vi "Host - LED encode (SubVI).vi"(7 "Address":u8, 9 "Dim Ctrl":u8, 10 "led":bool) -> (2 "string":string, 3 "Command":string)   [LabVIEW 2021]
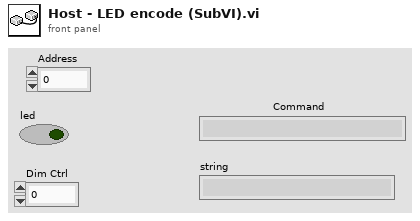
[diagram p1: front panel]
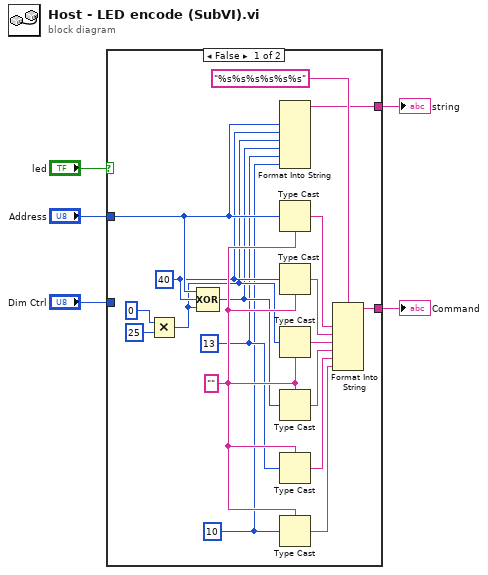
[diagram p0: block diagram]
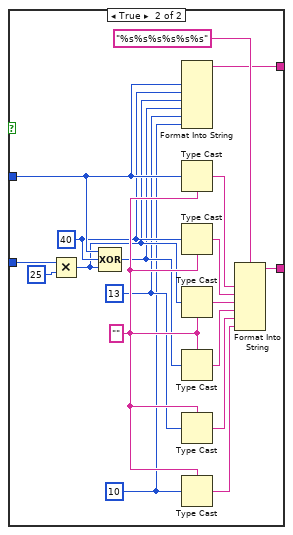
[diagram p2: hidden frame]
diagram:
  n1 = case shown="False" "led" {
    tunnel: "Dim Ctrl" -> [_ w41]
    tunnel: "Address" -> [w12 w30]
    tunnel: [w14 w31] -> w2
    tunnel: [w6 w24] -> w1
    frame False {
      w16 = "" ("type")
      w7 = u8 10 ("value")
      w8 = u8 13 ("value")
      w11 = u8 40 ("value")
      n2 = Multiply(x=u8 0, y=u8 25) -> (x*y=w10:u8)
      n3 = Compound Arithmetic op=XOR(w12, w11, w10) -> (w9:u8)
      n4 = Format Into String(w12, w11, w10, w9, w8, w7) -> (resulting string=w6:string)  [unwired: 3 in, 1 out]
      n5 = Type Cast(type=w16, x=w12) -> (*(type *) &x=w19:string)
      n6 = Type Cast(type=w16, x=w11) -> (*(type *) &x=w22:string)
      n7 = Type Cast(type=w16, x=w10) -> (*(type *) &x=w21:string)
      n8 = Type Cast(type=w16, x=w9) -> (*(type *) &x=w20:string)
      n9 = Type Cast(type=w16, x=w8) -> (*(type *) &x=w18:string)
      n10 = Type Cast(type=w16, x=w7) -> (*(type *) &x=w17:string)
      n11 = Format Into String(format string="%s%s%s%s%s%s", w19, w22, w21, w20, w18, w17) -> (resulting string=w14:string)  [unwired: 2 in, 1 out]
    }
    frame True {
      w32 = "" ("type")
      w25 = u8 10 ("value")
      w26 = u8 13 ("value")
      w29 = u8 40 ("value")
      n12 = Multiply(x=w41, y=u8 25) -> (x*y=w28:u8)
      n13 = Compound Arithmetic op=XOR(w30, w29, w28) -> (w27:u8)
      n14 = Format Into String(w30, w29, w28, w27, w26, w25) -> (resulting string=w24:string)  [unwired: 3 in, 1 out]
      n15 = Type Cast(type=w32, x=w30) -> (*(type *) &x=w35:string)
      n16 = Type Cast(type=w32, x=w29) -> (*(type *) &x=w38:string)
      n17 = Type Cast(type=w32, x=w28) -> (*(type *) &x=w37:string)
      n18 = Type Cast(type=w32, x=w27) -> (*(type *) &x=w36:string)
      n19 = Type Cast(type=w32, x=w26) -> (*(type *) &x=w34:string)
      n20 = Type Cast(type=w32, x=w25) -> (*(type *) &x=w33:string)
      n21 = Format Into String(format string="%s%s%s%s%s%s", w35, w38, w37, w36, w34, w33) -> (resulting string=w31:string)  [unwired: 2 in, 1 out]
    }
  }
  "Command" <- w2
  "string" <- w1
